vi "Clear.vi"(8 "error in (no error)":errorcluster, 11 "Process In":refnum<class "Debug Process.lvclass">) -> (0 "error out":errorcluster)   [LabVIEW 2020, in "Debug Process.lvclass"]
doc: "Clears any resorces allocated during initialization."
uses:
  Debug Process.lvclass
  Debug Process.lvclass/Debug Process.ctl
  <vilib>/Utility/error.llb/Clear Errors.vi
  <vilib>/Utility/error.llb/Error Cluster From Error Code.vi
  <vilib>/ErrorRing/Error Ring.xnode
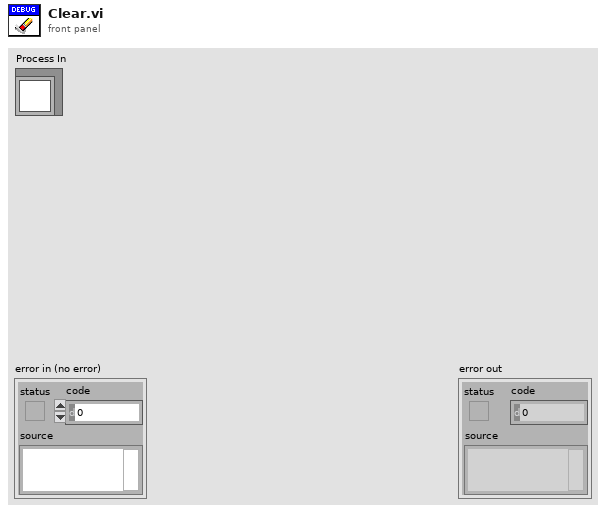
[diagram p1: front panel]
types:
  T1 = typedef "Debug Process.lvclass/Lifecycle State.ctl" = enum16{"Uninitialized", "Initialized", "Started", "Running", "Stopped", "Finished"}
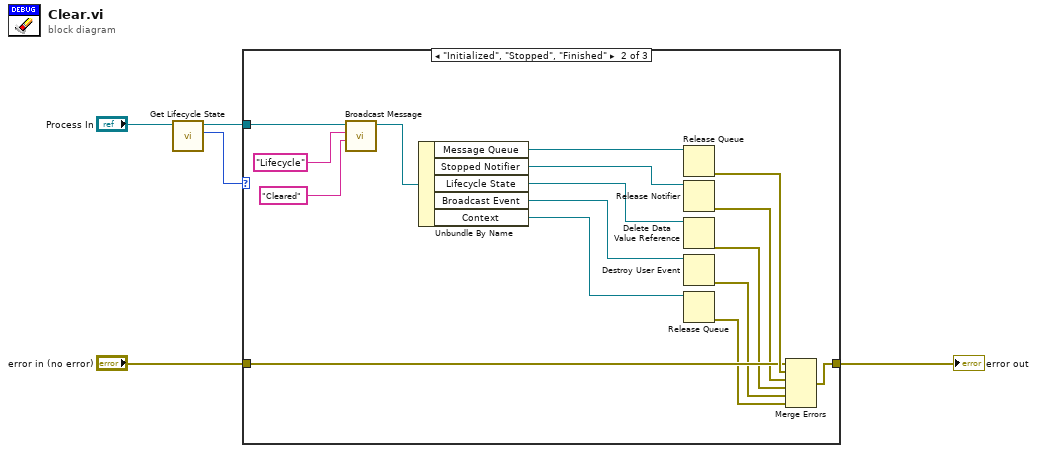
[diagram p0: block diagram]
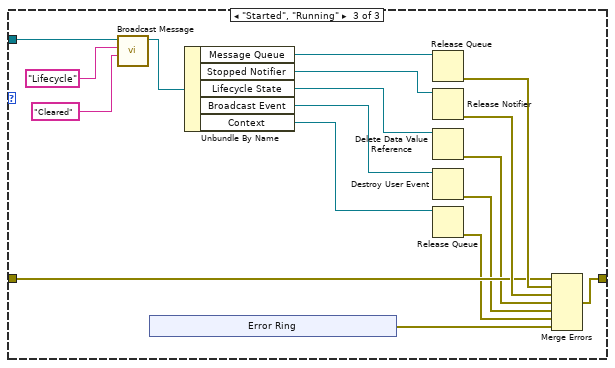
[diagram p3: hidden frame]
diagram:
  n1 = call "Get Lifecycle State.vi"("Process In"="Process In") -> ("Lifecycle State"=w3:T1, "Process Out"=w4:refnum<class "Debug Process.lvclass">)  [unwired: 7 in, 2 out]
  n2 = case shown="\"Initialized\", \"Stopped\", \"Finished\"" w3 {
    tunnel: [w6 w22 w39] -> w2
    tunnel: w4 -> [_ w7 w26]
    tunnel: "error in (no error)" -> [w6 w18 w34]
    frame "Uninitialized" {
    }
    frame "Initialized", "Stopped", "Finished" {
      n3 = call-dynamic "Broadcast Message.vi"("Message Data"="Cleared" ("Message"), "Message"="Lifecycle", "Process In"=w7) -> ("Process Out"=w8:refnum<class "Debug Process.lvclass">)  [unwired: 7 in, 1 out]
      n4 = Unbundle By Name(w8) -> ("Message Queue"=w21:refnum<queue>, "Stopped Notifier"=w19:refnum<notifier>, "Lifecycle State"=w17:refnum<data-value>, "Broadcast Event"=w15:refnum<user-event>, "Context"=w14:refnum<queue>)
      n5 = Release Queue(queue=w21) -> (error out=w20:errorcluster)  [unwired: 2 in, 2 out]
      n6 = Release Notifier(notifier=w19) -> (error out=w11:errorcluster)  [unwired: 2 in, 2 out]
      n7 = Delete Data Value Reference(data value reference=w17) -> (error out=w16:errorcluster)  [unwired: 1 in, 1 out]
      n8 = Destroy User Event(user event=w15) -> (error out=w13:errorcluster)  [unwired: 1 in]
      n9 = Release Queue(queue=w14) -> (error out=w12:errorcluster)  [unwired: 2 in, 2 out]
      n10 = Merge Errors(w18, w20, w11, w16, w13, w12) -> (w22:errorcluster)
    }
    frame "Started", "Running" {
      n11 = call-dynamic "Broadcast Message.vi"("Message Data"="Cleared" ("Message"), "Message"="Lifecycle", "Process In"=w26) -> ("Process Out"=w25:refnum<class "Debug Process.lvclass">)  [unwired: 7 in, 1 out]
      n12 = xnode "Error Ring"() -> ("error out"=w27:errorcluster)
      n13 = Unbundle By Name(w25) -> ("Message Queue"=w38:refnum<queue>, "Stopped Notifier"=w36:refnum<notifier>, "Lifecycle State"=w33:refnum<data-value>, "Broadcast Event"=w30:refnum<user-event>, "Context"=w29:refnum<queue>)
      n14 = Release Queue(queue=w38) -> (error out=w37:errorcluster)  [unwired: 2 in, 2 out]
      n15 = Release Notifier(notifier=w36) -> (error out=w35:errorcluster)  [unwired: 2 in, 2 out]
      n16 = Delete Data Value Reference(data value reference=w33) -> (error out=w32:errorcluster)  [unwired: 1 in, 1 out]
      n17 = Destroy User Event(user event=w30) -> (error out=w31:errorcluster)  [unwired: 1 in]
      n18 = Release Queue(queue=w29) -> (error out=w28:errorcluster)  [unwired: 2 in, 2 out]
      n19 = Merge Errors(w34, w37, w35, w32, w31, w28, w27) -> (w39:errorcluster)
    }
  }
  "error out" <- w2
